vi "Bulk Add AI Register - Right Click.vi"() -> ()   [LabVIEW 2015, in "Modbus Master System Explorer.lvlib"]
uses:
  Modbus Master System Explorer.lvlib
  <vilib>/NI Veristand/Custom Device API/Custom Device Item Ref.ctl
  Shared/Controls/Data Model/Mapping.ctl
  Shared/Controls/Data Model/DataType.ctl
  Shared/Modbus Master Shared.lvlib
  <vilib>/NI VeriStand/Custom Device API/Custom Device API.lvlib
panel:
  in  "Node Ptr":T1 format="%.0x"
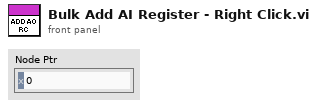
[diagram p1: front panel]
types:
  T1 = typedef "Custom Device API.lvlib/Custom Device Item Ref.ctl" = u64
  T2 = typedef "Modbus Master Shared.lvlib/DataType.ctl" = enum16{"Double", "Single", "I64", "I32", "I16", "I8", "U64", "U32", "U16", "U8", "Boolean"}
  T3 = typedef "Modbus Master Shared.lvlib/Mapping.ctl" = cluster{"DataType":T2, "Starting Address":u16, "Sub-Index (Bool)":u16, "VS Reference":T1}
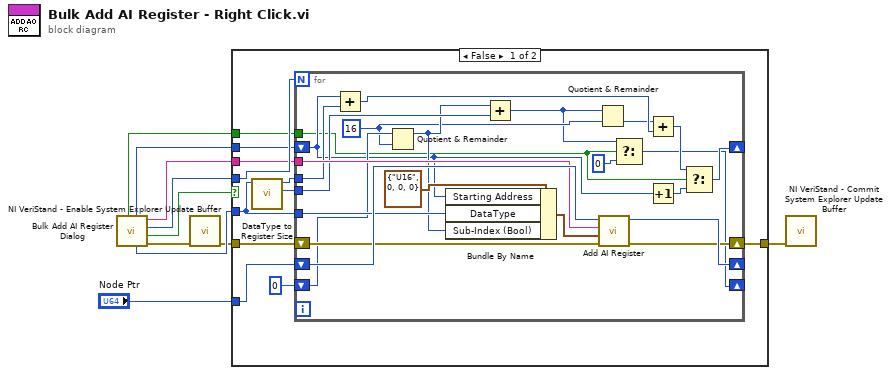
[diagram p0: block diagram]
diagram:
  n1 = call "Bulk Add AI Register Dialog.vi"() -> ("error out"=w2:errorcluster, "Cancelled?"=w7:bool, "Quantity Out"=w8:u16, "Root Name Out"=w9:string, "DataType Out"=w6:T2, "Starting Address Out"=w10:u16, "Pack Values? Out"=w4:bool)  [unwired: 5 in]
  n2 = call <vilib>:"NI VeriStand - Enable System Explorer Update Buffer.vi"("error in (no error)"=w2) -> ("error out"=w1:errorcluster)  [unwired: 10 in]
  n3 = case shown="False" w7 {
    tunnel: "Node Ptr" -> [w14 _]
    tunnel: w8 -> [w21 _]
    tunnel: w1 -> [w15 w45]
    tunnel: w9 -> [w20 _]
    tunnel: w10 -> [w19 _]
    tunnel: w6 -> [w13 _]
    tunnel: w4 -> [w12 _]
    tunnel: [w11 w45] -> w3
    frame False {
      n4 = call "DataType to Register Size.vi"("DataType"=w13) -> ("bits"=w16:i32, "bytes"=w18:i32)  [unwired: 9 in]
      n5 = for {
        N: w21 -> [_]
        shift-right: [w42] -> _
        shift-left: w14 -> [w44]
        shift-right: [w40] -> w11
        shift-left: w15 -> [w43]
        tunnel: w20 -> [w41]
        shift-right: [w27] -> _
        shift-left: w19 -> [w29]
        tunnel: w13 -> [w38]
        tunnel: w18 -> [w37]
        shift-right: [w24] -> _
        shift-left: 0 ("Sub-Index (Bool)") -> [w35]
        tunnel: w16 -> [w36]
        tunnel: w12 -> [w26]
        w32 = 16 ("y")
        n6 = Add(x=w29, y=w37) -> (x+y=w33:i32)
        n7 = Quotient & Remainder(x=w35, y=w32) -> (x-y*floor(x/y)=w34:i32)  [unwired: 1 out]
        n8 = Bundle By Name(cluster=T3 {"DataType"=enum."U16", "Starting Address"=0, "Sub-Index (Bool)"=0, "VS Reference"=0} ("Mapping"), "Starting Address"=w29, "DataType"=w38, "Sub-Index (Bool)"=w34) -> (w22:T3)
        n9 = Add(x=w34, y=w36) -> (x+y=w25:i32)
        n10 = Quotient & Remainder(x=w25, y=w32) -> (floor(x/y)=w31:i32)  [unwired: 1 out]
        n11 = call "Add AI Register.vi"("error in (no error)"=w43, "Mapping"=w22, "Label"=w41, "Node Ref In"=w44) -> ("error out"=w40:errorcluster, "Node Ref out"=w42:T1)  [unwired: 5 in, 1 out]
        n12 = Select(t=w25, s=w26, f=0 ("t")) -> (s? t:f=w24:i32)
        n13 = Add(x=w31, y=w33) -> (x+y=w28:i32)
        n14 = Increment(x=w29) -> (x+1=w30:i32)
        n15 = Select(t=w28, s=w26, f=w30) -> (s? t:f=w27:i32)
      }
    }
    frame True {
    }
  }
  n16 = call <vilib>:"NI VeriStand - Commit System Explorer Update Buffer.vi"("error in (no error)"=w3) -> ()  [unwired: 10 in, 1 out]
